vi "MHL Queue Ref Holder.vi"(6 "Action":enum16{"GET", "SET"}(ring), 8 "error in":errorcluster, 11 "Message Queue In":refnum<queue>) -> (0 "error out":errorcluster, 3 "Input Message Queue":refnum<queue>)   [LabVIEW 2015]
doc: "Holds UI queue reference to enqueue messages without wiring"
uses:
  Message Queue/Message Cluster.ctl
  Message Queue/Message Queue.lvlib
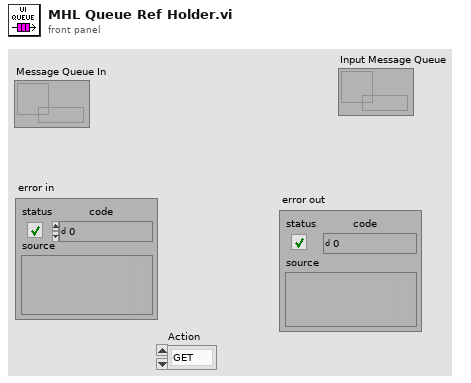
[diagram p1: front panel]
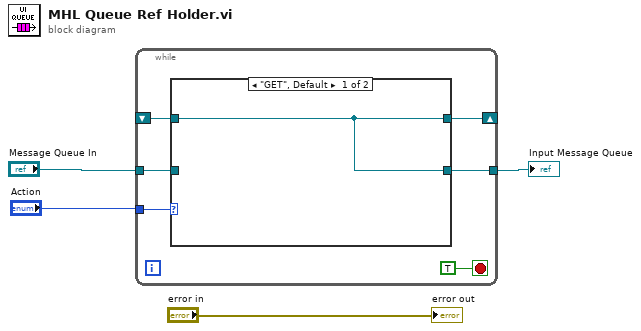
[diagram p0: block diagram]
diagram:
  n1 = while {
    tunnel: "Message Queue In" -> [w9]
    tunnel: [w5] -> w3
    tunnel: "Action" -> [w6]
    shift-right: [w8] -> _
    shift-left: _ -> [w7]
    stop <- TRUE stop-if-true
    n2 = case shown="\"GET\", Default" w6 {
      tunnel: w9 -> [_ w12]
      tunnel: [w11 w12] -> w8
      tunnel: w7 -> [w11 _]
      tunnel: [w11 w12] -> w5
      frame "GET", Default {
      }
      frame "SET" {
      }
    }
  }
  "Input Message Queue" <- w3
  "error out" <- "error in"
